vi "Stop Core.vi"(10 "final error code":i32, 11 "Display_Console in":refnum<class "Display_Console.lvclass">) -> (3 "Display_Console out":refnum<class "Display_Console.lvclass">)   [LabVIEW 2025, in "Display_Console.lvlib" / "Display_Console.lvclass"]
doc: "<p>(<strong>Filename</strong>: <span class=\"dnl\">Actor Framework.lvlib:Actor.lvclass:Stop Core.vi</span>)</p>\n<p>Defines what the actor does before it stops. Use the <strong>final error code</strong> input to determine whether the actor shut down in response to an error.</p>\n<p>By default, this method passes the Stop message along to all <a href=\"nihelplauncher://docs/csh?context=lvcore_lvcomm_af_launch_nested_actor\">auto-stop nested actors</a>. A descendant class may override this method to define additional behavior, such as shutting down any processes the actor initiated in its override of the <a href=\"nihelplauncher://docs/csh?context=lvcore_lvcomm_af_actor_core\">Actor Core</a> method.</p>"
uses:
  Display_Console.lvclass
  Display_Console.lvclass/Display_Console.ctl
  <vilib>/ni/Actors/State Actor/State Actor/State Actor.lvclass
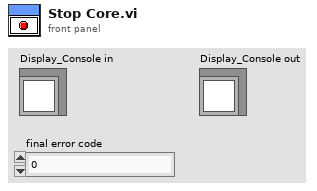
[diagram p1: front panel]
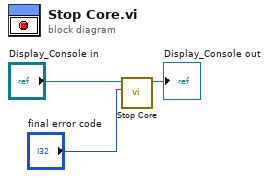
[diagram p0: block diagram]
diagram:
  n1 = call-parent "Stop Core.vi"("final error code"="final error code", "Actor in"="Display_Console in") -> ("Actor out"=→"Display_Console out":refnum<class "Display_Console.lvclass">)  [unwired: 9 in]
